vi "testPeriodicStateStringDoStateNow.vi"(8 "error in (no error)":errorcluster, 11 "testStateMachineUtilities in":refnum<class "testStateMachineUtilities.lvclass">) -> (0 "error out":errorcluster, 3 "testStateMachineUtilities out":refnum<class "testStateMachineUtilities.lvclass">)   [LabVIEW 2013, in "testStateMachineUtilities.lvclass"]
uses:
  testStateMachineUtilities.lvclass
  source/State Machine Support API/Conditional State String.vi
  <userlib>/_OpenG.lib/time/time.llb/Periodic Trigger__ogtk.vi
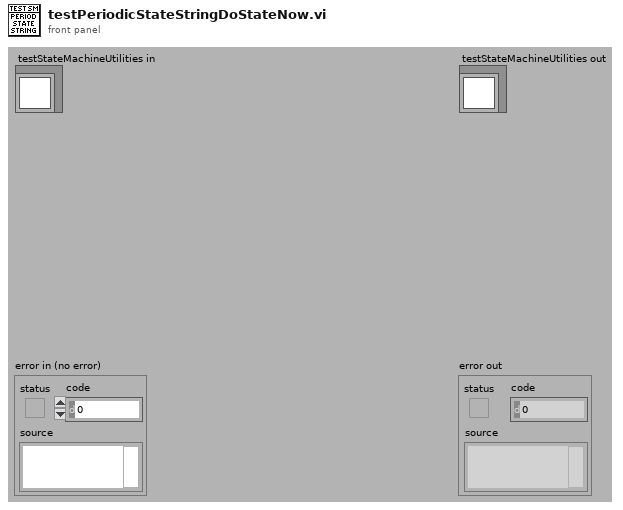
[diagram p1: front panel]
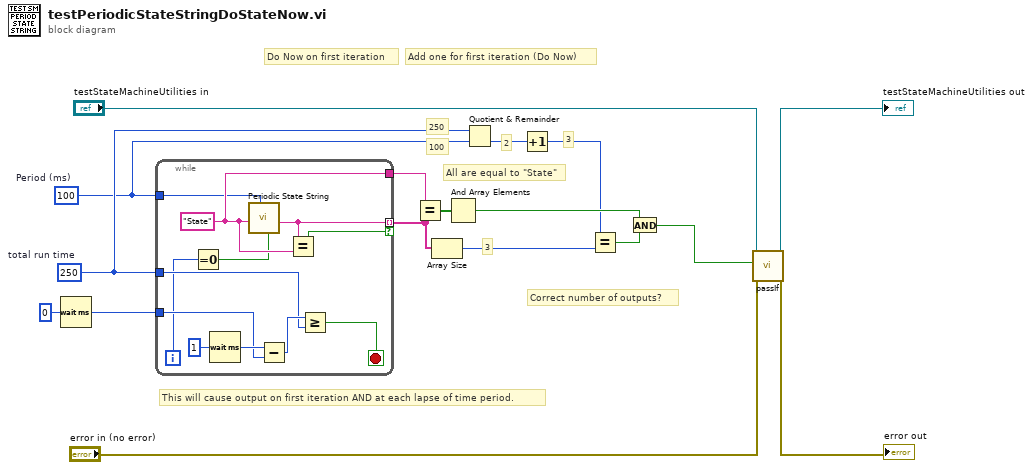
[diagram p0: block diagram]
diagram:
  w7 = u32 100  # Period (ms)
  w8 = u32 250  # total run time
  # "This will cause output on first iteration AND at each lapse of time period."
  # "3"
  # "Do Now on first iteration"
  # "Add one for first iteration (Do Now)"
  # "Correct number of outputs?"
  # "3"
  # "2"
  # "100"
  # "250"
  # "All are equal to \"State\""
  n1 = Wait (ms)(milliseconds to wait=u32 0) -> (millisecond timer value=w12:u32)
  n2 = while {
    tunnel: [w29] -> w9 mode=indexing if=w28
    tunnel: w12 -> [w25]
    tunnel: w8 -> [w21]
    tunnel: [w24] -> w11
    tunnel: w7 -> [w23]
    i -> [w19]
    stop <- w20 stop-if-true
    w24 = "State" ("State Queue")
    n3 = Equal To 0?(x=w19) -> (x = 0?=w18:bool)
    n4 = Wait (ms)(milliseconds to wait=u32 1) -> (millisecond timer value=w26:u32)
    n5 = call "Periodic State String.vi"("Do State Now? (Reset Period)"=w18, "Period (ms)"=w23, "State"=w24) -> ("State Out"=w29:string)  [unwired: 8 in]
    n6 = Subtract(x=w26, y=w25) -> (x-y=w22:u32)
    n7 = Equal?(x=w29, y=w24) -> (x = y?=w28:bool)
    n8 = Greater Or Equal?(x=w22, y=w21) -> (x >= y?=w20:bool)
  }
  n9 = Equal?(x=w11, y=w9) -> (x = y?=w10:bool[])
  n10 = Array Size(array=w9) -> (size(s)=w5:i32)
  n11 = And Array Elements(Boolean array=w10) -> (logical AND=w3:bool)
  n12 = Quotient & Remainder(x=w8, y=w7) -> (floor(x/y)=w6:u32)  [unwired: 1 out]
  n13 = Increment(x=w6) -> (x+1=w1:u32)
  n14 = Equal?(x=w1, y=w5) -> (x = y?=w4:bool)
  n15 = And(x=w3, y=w4) -> (x .and. y?=w2:bool)
  n16 = call-dynamic "passIf.vi"("error in (no error)"="error in (no error)", "pass"=w2, "TestCase in"="testStateMachineUtilities in") -> ("error out"=→"error out":errorcluster, "TestCase out"=→"testStateMachineUtilities out":refnum<class "testStateMachineUtilities.lvclass">)  [unwired: 7 in]
